vi "CleanUp.vi"(0 "object in":refnum<class "Fuente de poder.lvclass">, 5 "error in (no error)":errorcluster) -> (14 "object out":refnum<class "Fuente de poder.lvclass">, 19 "error out":errorcluster)   [LabVIEW 2020, in "Fuente de poder.lvclass"]
uses:
  Fuente de poder.lvclass
  Fuente de poder.lvclass/Fuente de poder.ctl
  Instrumento/Instrumento.lvclass
  <resource>/Framework/Providers/Open_GDS/ClassProviders/Provider_LvNativeClass/Templates/NativeSubTemplate/NativeSubTemplate.lvclass
  C:/Program Files (x86)/National Instruments/LabVIEW 2020/resource/Framework/Providers/Open_GDS/ClassProviders/Provider_LvNativeClass/Templates/NativeBaseTemplate/NativeBaseTemplate.lvclass
  C:/Program Files (x86)/National Instruments/LabVIEW 2020/resource/Framework/Providers/Open_GDS/ClassProviders/Provider_LvNativeClass/Templates/NativeSubTemplate/NativeSubTemplate.lvclass
  D:/Storage/Source Code/Clase AF/ClaseAF/11 OOP Interfaces/Instrumento/Instrumento.lvclass
  D:/Storage/Source Code/Clase AF/ClaseAF/11 OOP Interfaces/Fuente de poder_class/Fuente de poder.lvclass
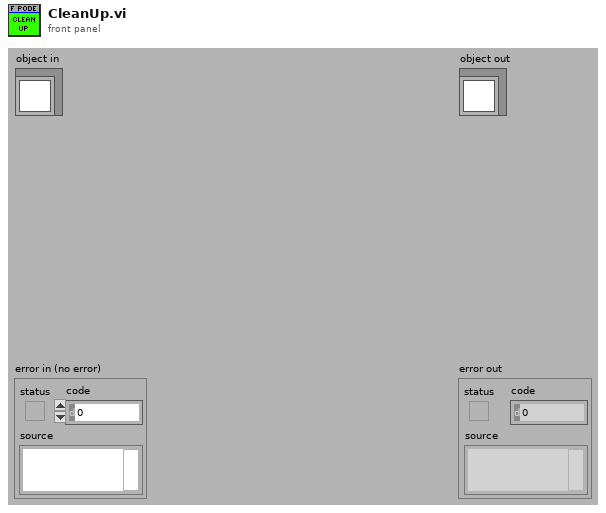
[diagram p1: front panel]
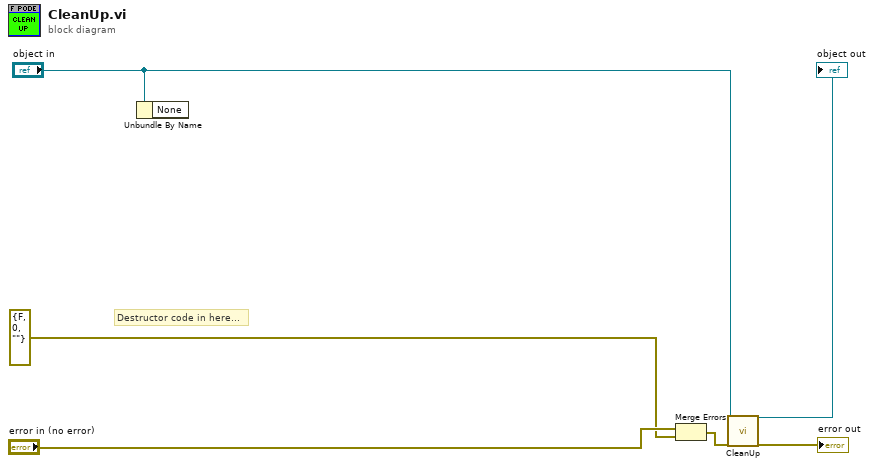
[diagram p0: block diagram]
diagram:
  # "Destructor code in here..."
  n1 = Unbundle By Name("object in") -> ()  [unwired: 1 out]
  n2 = Merge Errors("error in (no error)", errorcluster {"status"=FALSE, "code"=0, "source"=""} ("error in (no error)")) -> (w4:errorcluster)
  n3 = call-parent "CleanUp.vi"("object in"="object in", "error in (no error)"=w4) -> ("object out"=→"object out":refnum<class "NativeSubTemplate.lvclass">, "error out"=→"error out":errorcluster)  [unwired: 16 in]
